vi "Configure Extern Program Channel MX.vi"(0 "VISA resource name":refnum<visa-resource-name>, 1 "Channel":u8=1 min=1 max=3 step=1, 2 "Value":dbl min=-9000.0 max=9000.0, 3 "error in":errorcluster) -> (7 "VISA resource name out":refnum<visa-resource-name>, 10 "error out":errorcluster)   [LabVIEW 2015, in "IT-M3900C.lvlib"]
doc: "This command sets the linear calibration coefficients for channels (1/2/3).This instruction needs to set two parameters, separated by a comma, with the channel number in front of the comma and the linear calibration coefficient behind the comma.\n<b>Channel</b>\n1-3\n<b>Value</b>\n-9000~9000"
uses:
  <instrlib>/IT-M3900C/IT-M3900C.lvlib
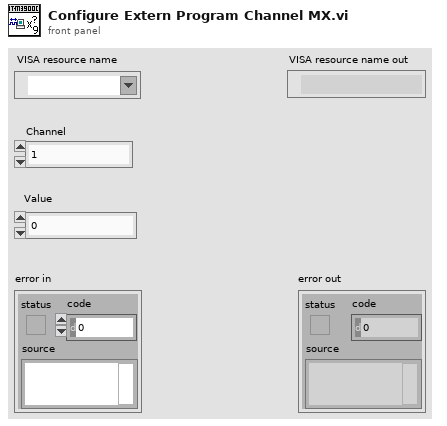
[diagram p1: front panel]
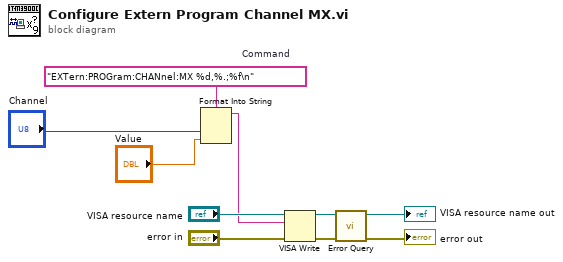
[diagram p0: block diagram]
diagram:
  w4 = "EXTern:PROGram:CHANnel:MX %d,%.;%f\n"  # Command
  n1 = Format Into String(format string=w4, "Channel", "Value") -> (resulting string=w3:string)  [unwired: 2 in, 1 out]
  n2 = VISA Write(VISA resource name="VISA resource name", write buffer=w3, error in (no error)="error in") -> (VISA resource name out=w7:refnum<visa-resource-name>, error out=w8:errorcluster)  [unwired: 1 out]
  n3 = call <instrlib>:"Error Query.vi"("error in"=w8, "VISA resource name"=w7) -> ("error out"=→"error out":errorcluster, "VISA resource name out"=→"VISA resource name out":refnum<visa-resource-name>)  [unwired: 6 in, 2 out]
